vi "XBee_UART_Setup_TX.vi"(8 "error in (no error)":errorcluster, 10 "Characters to Write":string, 11 "VISA resource name in":refnum<visa-resource-name>="ASRL1::INSTR") -> (0 "error out":errorcluster)   [LabVIEW 2018]
uses:
  <vilib>/myRIO/Instrument Drivers/Onboard IO/UART/typedef/VISA Configuration.ctl
  <vilib>/Instr/_visa.llb/VISA Configure Serial Port (Instr).vi
  <vilib>/myRIO/Instrument Drivers/Onboard IO/UART/UART.lvlib
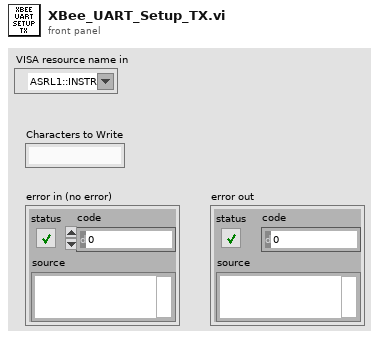
[diagram p1: front panel]
types:
  T1 = typedef "UART.lvlib/VISA Configuration.ctl" = cluster{"baud rate (9600)":u32, "data bits (8)":u16, "parity (0:none)":enum16{"None", "Odd", "Even", "Mark", "Space"}, "stop bits (10: 1 bit)":u16, "flow control (0:none)":u16, "termination char\n(0xA = '\\n' = LF) ":u8, "Enable Termination\nChar (T)":bool, "timeout (10sec)":u32}
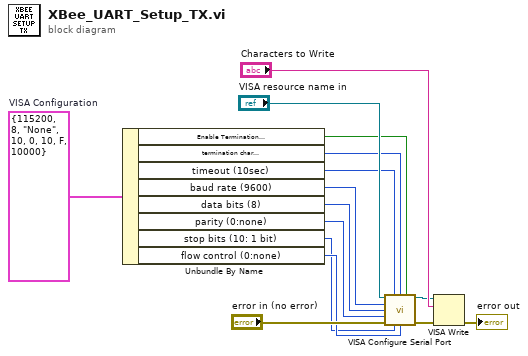
[diagram p0: block diagram]
diagram:
  w14 = T1 {"baud rate (9600)"=115200, "data bits (8)"=8, "parity (0:none)"=enum."None", "stop bits (10: 1 bit)"=10, "flow control (0:none)"=0, "termination char\n(0xA = '\\n' = LF) "=10, "Enable Termination\nChar (T)"=FALSE, "timeout (10sec)"=10000}  # VISA Configuration
  n1 = Unbundle By Name(w14) -> ("Enable Termination\nChar (T)"=w8:bool, "termination char\n(0xA = '\\n' = LF)"=w7:u8, "timeout (10sec)"=w6:u32, "baud rate (9600)"=w1:u32, "data bits (8)"=w2:u16, "parity (0:none)"=w3:enum16{"None", "Odd", "Even", "Mark", "Space"}, "stop bits (10: 1 bit)"=w4:u16, "flow control (0:none)"=w5:u16)
  n2 = call-poly "VISA Configure Serial Port"("VISA resource name"="VISA resource name in", "timeout (10sec)"=w6, "termination char\n(0xA = '\\n' = LF)"=w7, "Enable Termination\nChar (T)"=w8, "baud rate (9600)"=w1, "data bits (8)"=w2, "parity (0:none)"=w3, "error in (no error)"="error in (no error)", "stop bits (10: 1 bit)"=w4, "flow control (0:none)"=w5) -> ("VISA resource name out"=w11:refnum<visa-resource-name>, "error out"=w10:errorcluster)  [unwired: 4 in]
  n3 = VISA Write(VISA resource name=w11, write buffer="Characters to Write", error in (no error)=w10) -> (error out=→"error out":errorcluster)  [unwired: 2 out]
